vi "I2C_Download.vi"(11 "newFlashFW":u8[](array[numeric])) -> ()   [LabVIEW 2016]
uses:
  Global variable.vi
panel:
  out "status":u8
  in  "cmd_std_header_t":T1
  in  "执行部分":T2(ring)
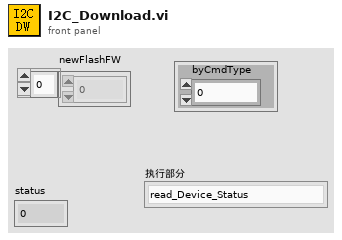
[diagram p1: front panel]
types:
  T1 = cluster{"byCmdType":u8, "bySubCmd":u8, "byPara":u8, "byAddr_h":u8, "byAddr_l":u8, "byAddr_ll":u8, "byLen_h":u8, "byLen_l":u8}
  T2 = enum16{"read_Device_Status", "RST_2_updateFW", "read_flashID_and_reset_flash", "erase_flash", "erase_check", "update_flashFW", "read_and_check", "write_Cache_TAG", "RST_2_ROM_and_check"}
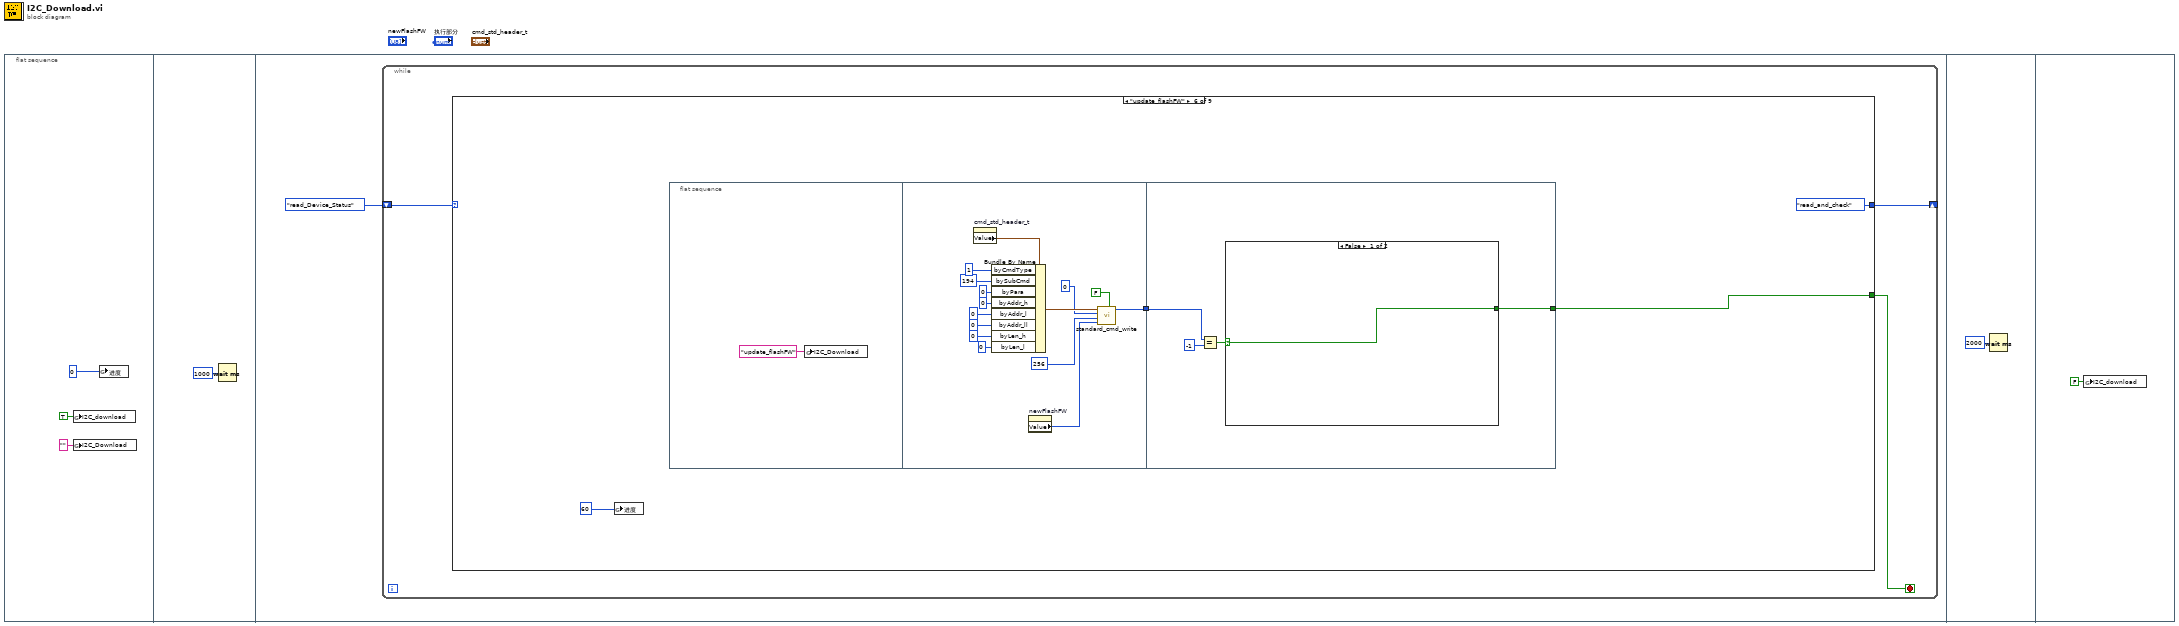
[diagram p0: block diagram]
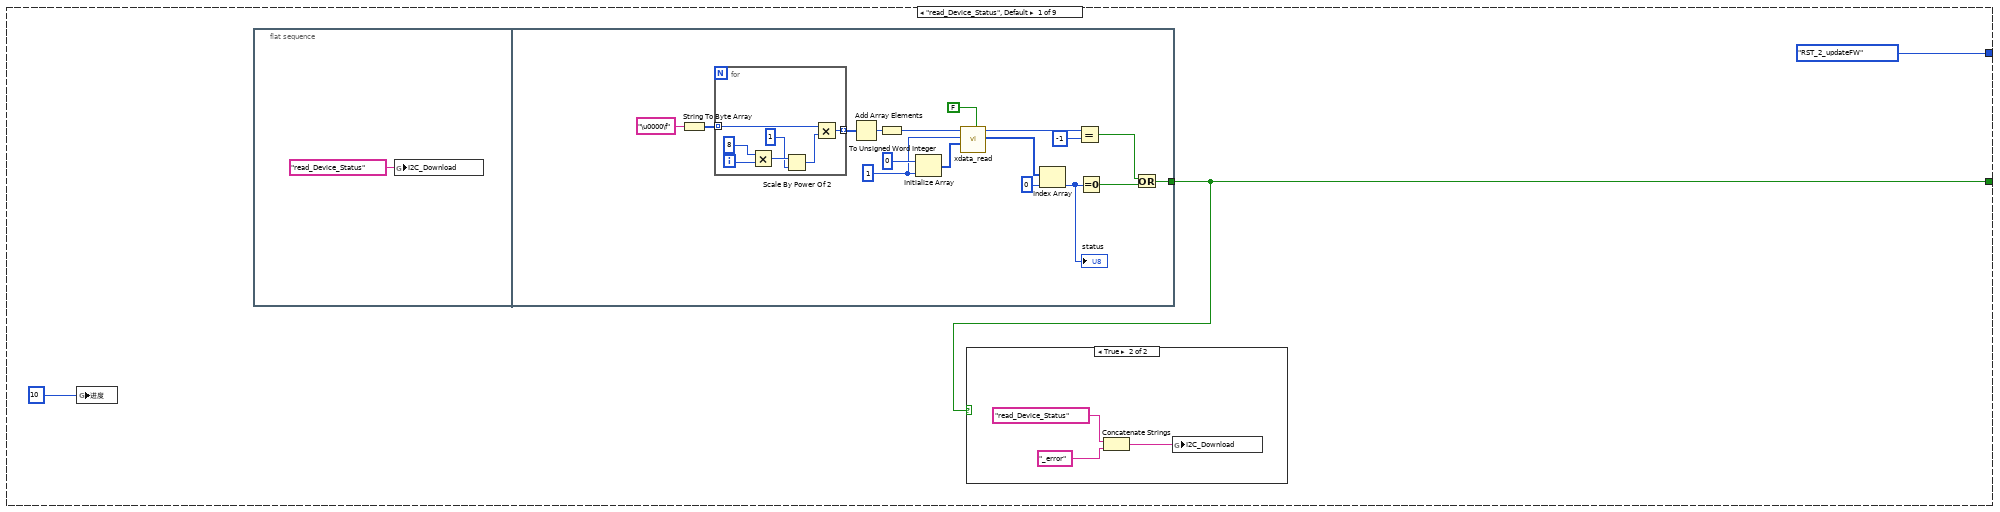
[diagram p2: hidden frame]
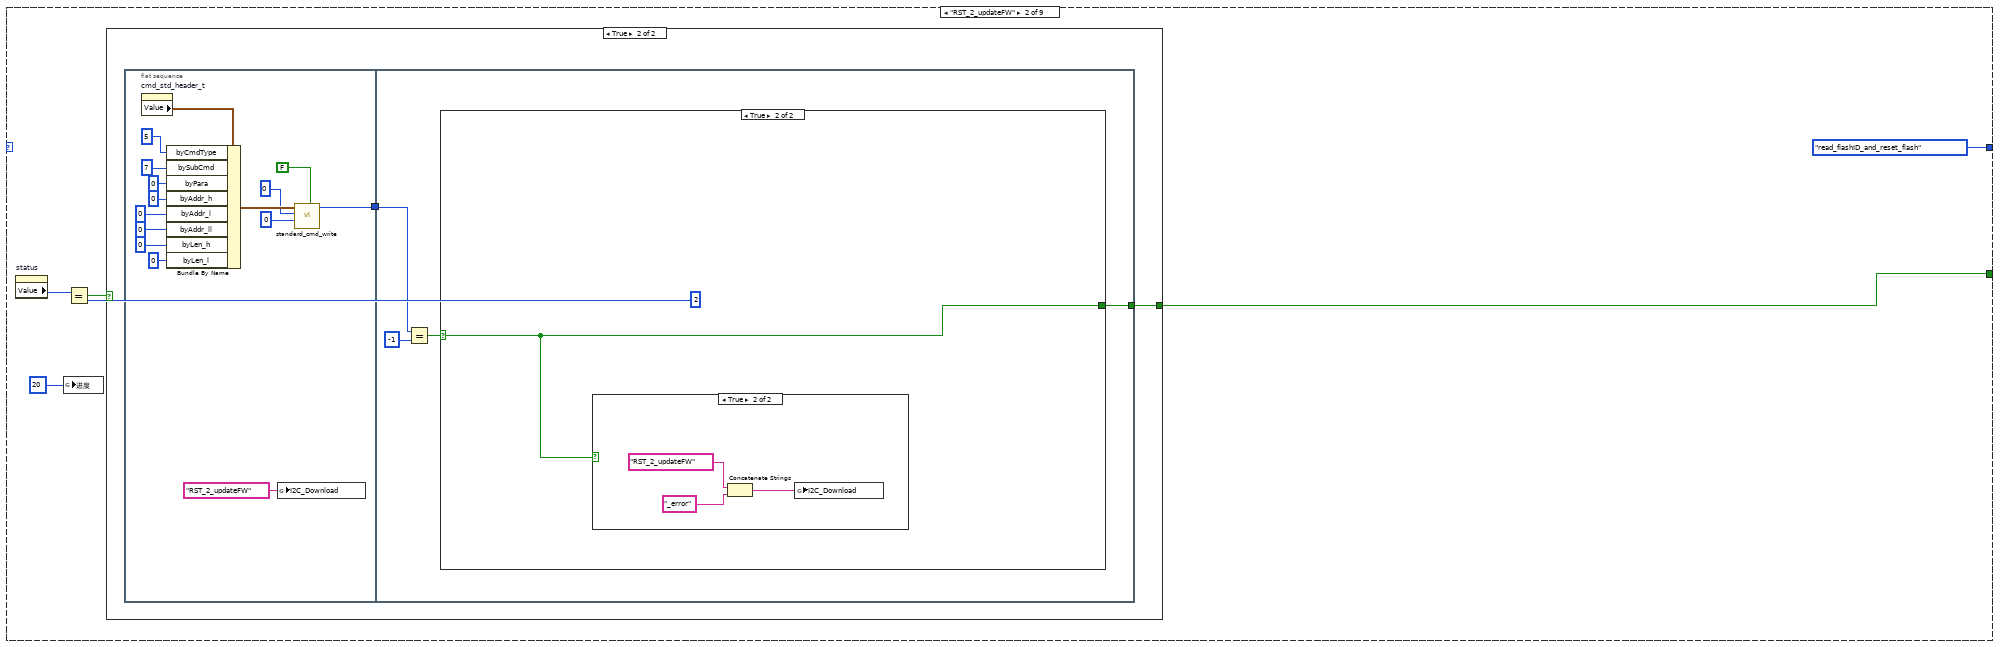
[diagram p4: hidden frame]
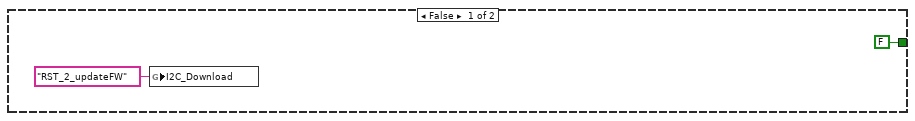
[diagram p5: hidden frame]
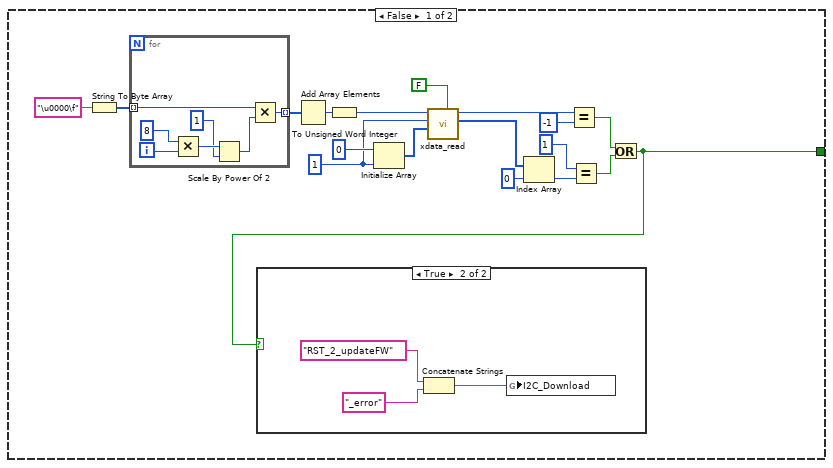
[diagram p6: hidden frame]
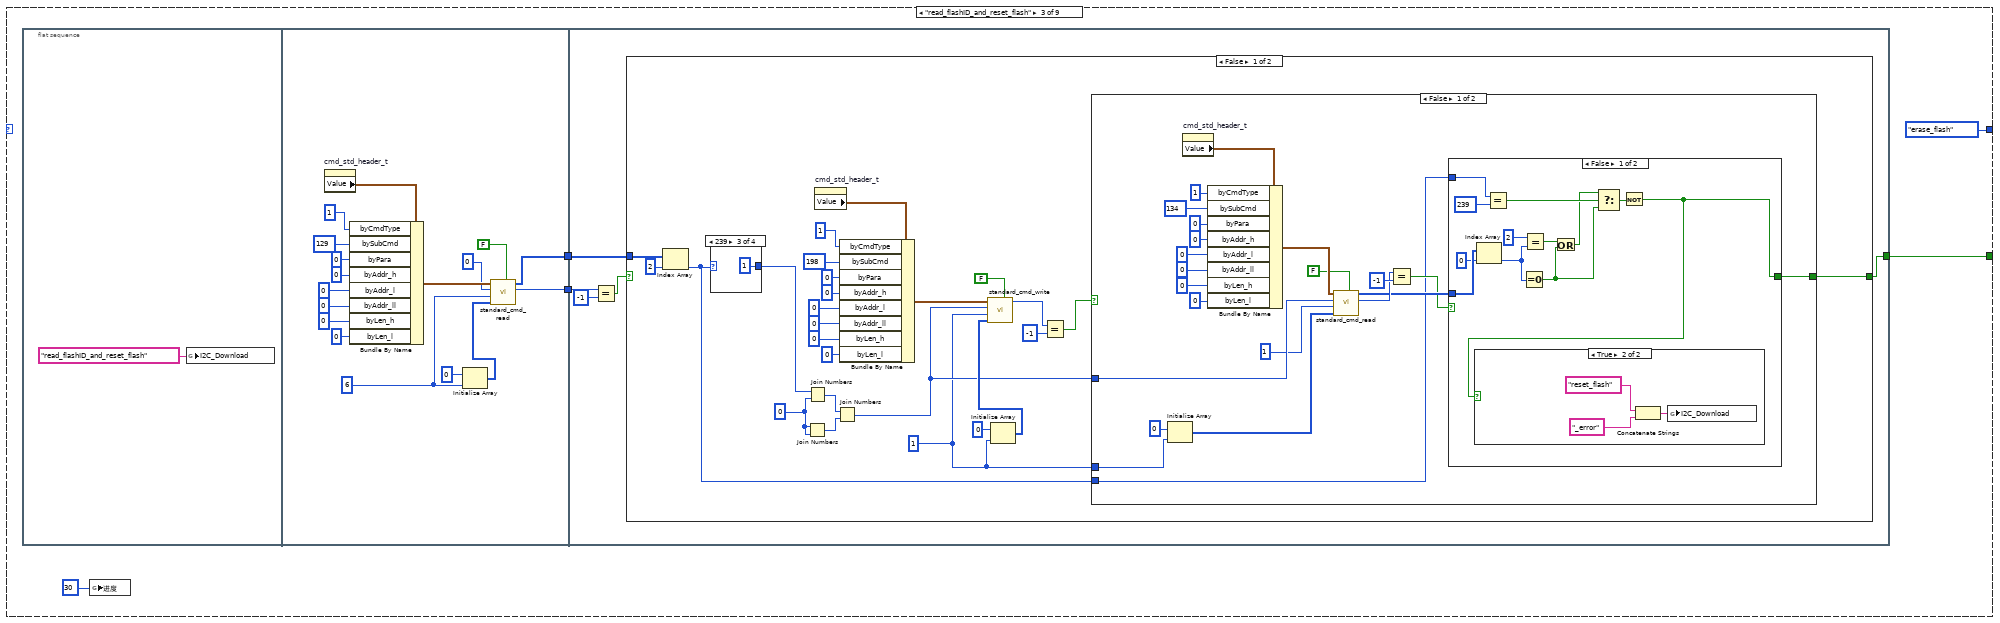
[diagram p9: hidden frame]
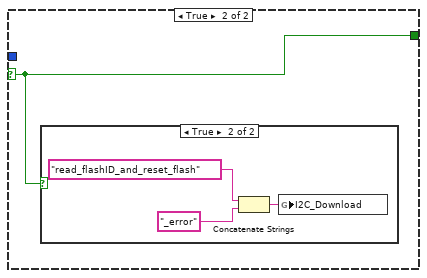
[diagram p11: hidden frame]
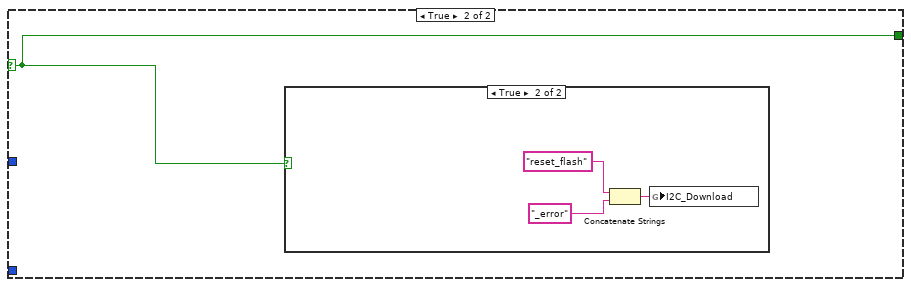
[diagram p13: hidden frame]
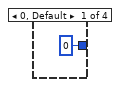
[diagram p15: hidden frame]
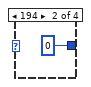
[diagram p16: hidden frame]
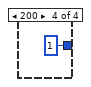
[diagram p17: hidden frame]
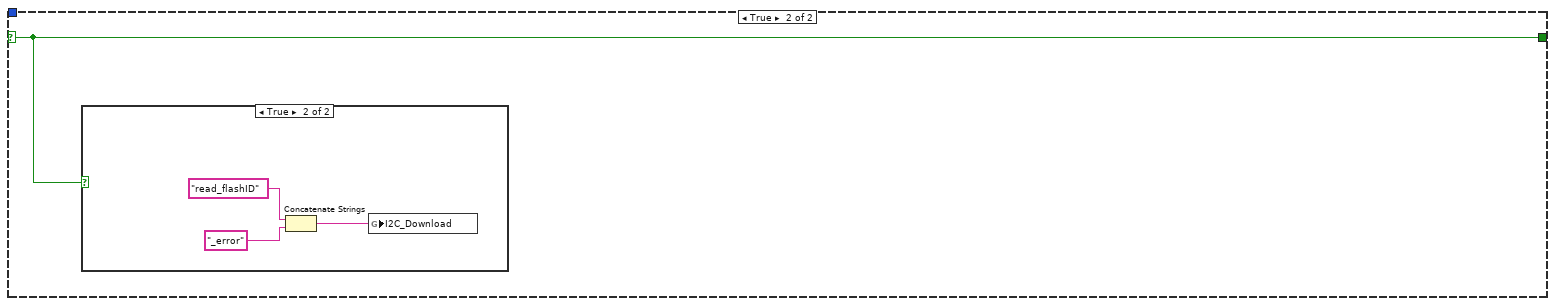
[diagram p18: hidden frame]
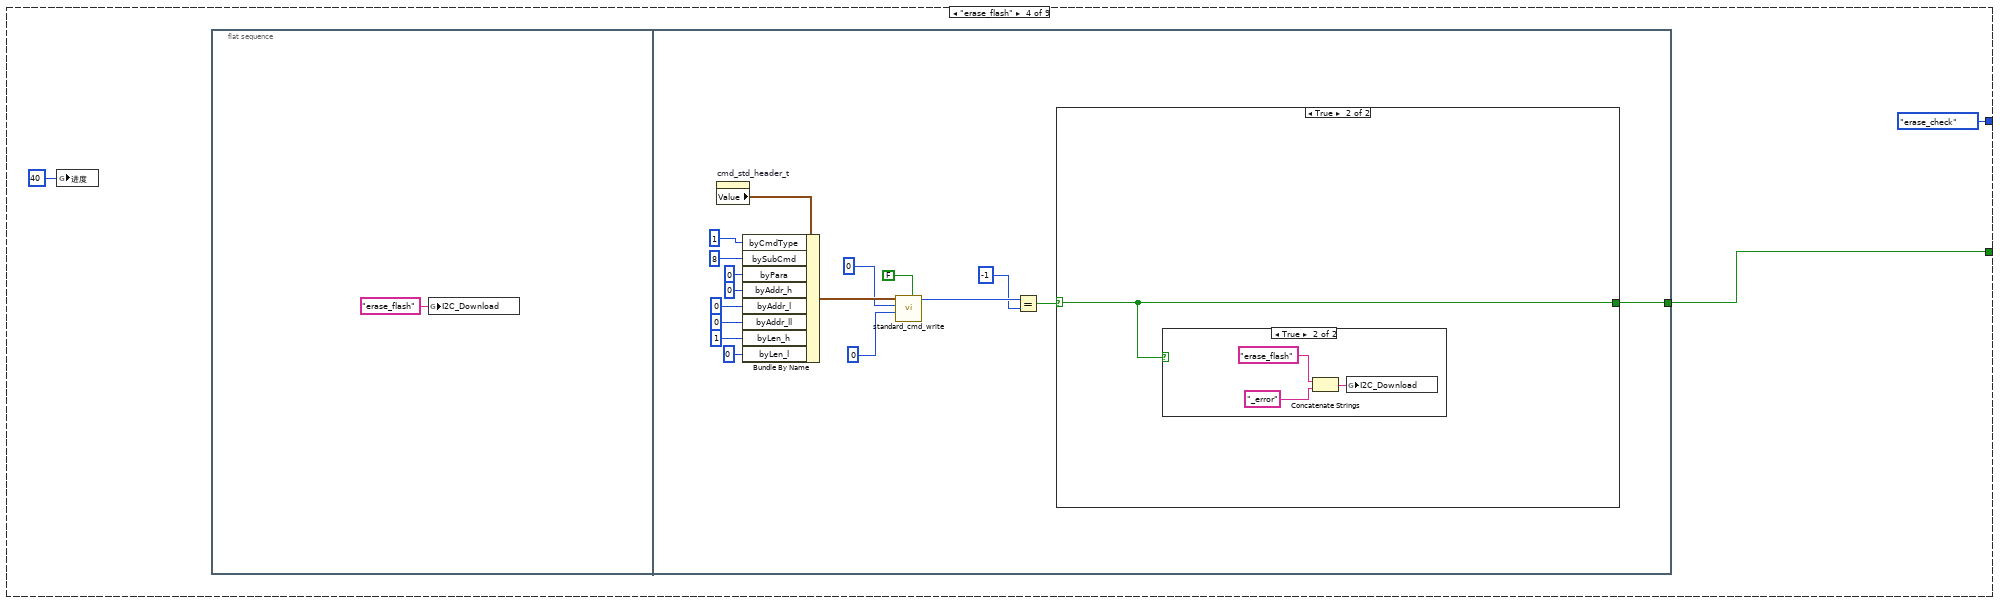
[diagram p20: hidden frame]
diagram:
  n1 = flat-sequence {
    frame #0 {
      n2 = global write "Global variable.vi" "I2C_download"(TRUE ("I2C_download")) -> ()
      n3 = global write "Global variable.vi" "I2C_Download"("" ("I2C_Download")) -> ()
      n4 = global write "Global variable.vi" "进度"(u8 0 ("进度")) -> ()
    }
    frame #1 {
      n5 = Wait (ms)(milliseconds to wait=u32 1000) -> ()  [unwired: 1 out]
    }
    frame #2 {
      n6 = while {
        shift-right: [w7] -> _
        shift-left: T2."read_Device_Status" ("执行部分") -> [w8]
        stop <- w6 stop-if-true
        n7 = case shown="\"update_flashFW\"" w8 {
          tunnel: [T2."RST_2_updateFW" ("执行部分") T2."read_flashID_and_reset_flash" ("执行部分") T2."erase_flash" ("执行部分") T2."erase_check" ("执行部分") T2."update_flashFW" ("执行部分") T2."read_and_check" ("执行部分") T2."write_Cache_TAG" ("执行部分") T2."RST_2_ROM_and_check" ("执行部分") T2."read_Device_Status" ("执行部分")] -> w7
          tunnel: [w10 w41 w102 w210 w236 w310 w339 w383 w411] -> w6
          frame "read_Device_Status", Default {
            n8 = global write "Global variable.vi" "进度"(u8 10 ("进度")) -> ()
            n9 = flat-sequence {
              tunnel: [w16] -> w10
              frame #0 {
                n10 = global write "Global variable.vi" "I2C_Download"("read_Device_Status" ("I2C_Download")) -> ()
              }
              frame #1 {
                w25 = 1 ("dimension size")
                n11 = String To Byte Array(string="\u0000\f") -> (unsigned byte array=w31:u8[])
                n12 = for {
                  tunnel: w31 -> [w34] mode=indexing
                  tunnel: [w33] -> w29 mode=indexing
                  i -> [w39]
                  n13 = Multiply(x=8, y=w39) -> (x*y=w37:i32)
                  n14 = Scale By Power Of 2(n=w37, x=1 ("x*y")) -> (x*2^n=w35:i32)
                  n15 = Multiply(x=w34, y=w35) -> (x*y=w33:i32)
                }
                n16 = Add Array Elements(numeric array=w29) -> (sum=w32:i32)
                n17 = To Unsigned Word Integer(number=w32) -> (unsigned 16bit integer=w28:u16)
                n18 = Initialize Array(u8 0 ("element"), w25) -> (w26:u8[])
                n19 = call "xdata_read.vi"("COM"=FALSE, "data"=w26, "wLen"=w25, "wAddr"=w28) -> ("data out"=w23:u8[], "return"=w20:i32)  [unwired: 6 in]
                n20 = Index Array(array=w23, index=0) -> (element=w21:u8)
                "status" <- w21
                n21 = Equal?(x=w20, y=-1) -> (x = y?=w18:bool)
                n22 = Equal To 0?(x=w21) -> (x = 0?=w17:bool)
                n23 = Or(x=w18, y=w17) -> (x .or. y?=w16:bool)
              }
            }
            n24 = case shown="True" w10 {
              frame False {
              }
              frame True {
                n25 = Concatenate Strings("read_Device_Status" ("I2C_Download"), "_error" ("I2C_Download")) -> (w12:string)
                n26 = global write "Global variable.vi" "I2C_Download"(w12) -> ()
              }
            }
          }
          frame "RST_2_updateFW" {
            n27 = property on="status" class="DigNum (strict)"() -> ("Value"=w45:u8)  [unwired: 2 in, 2 out]
            n28 = global write "Global variable.vi" "进度"(u8 20 ("进度")) -> ()
            n29 = Equal?(x=w45, y=u8 2) -> (x = y?=w43:bool)
            n30 = case shown="True" w43 {
              tunnel: [FALSE w48] -> w41
              frame False {
                n31 = global write "Global variable.vi" "I2C_Download"("RST_2_updateFW" ("I2C_Download")) -> ()
              }
              frame True {
                n32 = flat-sequence {
                  tunnel: [w51] -> w49
                  tunnel: w49 -> [w67]
                  tunnel: [w65] -> w48
                  frame #0 {
                    n33 = property on="cmd_std_header_t" class="Clust (strict)"() -> ("Value"=w64:T1)  [unwired: 2 in, 2 out]
                    n34 = Bundle By Name(cluster=w64, "byCmdType"=u8 5, "bySubCmd"=u8 7, "byPara"=u8 0, "byAddr_h"=u8 0, "byAddr_l"=u8 0, "byAddr_ll"=u8 0, "byLen_h"=u8 0, "byLen_l"=u8 0) -> (w55:T1)
                    n35 = global write "Global variable.vi" "I2C_Download"("RST_2_updateFW" ("I2C_Download")) -> ()
                    n36 = call "standard_cmd_write.vi"("COM"=FALSE, "dwLen"=u32 0, "dwAddr"=u32 0, "cmd_std_header_t"=w55) -> ("return"=w51:i32)  [unwired: 7 in]
                  }
                  frame #1 {
                    n37 = Equal?(x=w67, y=-1) -> (x = y?=w68:bool)
                    n38 = case shown="True" w68 {
                      selector: w68 -> [_ w97]
                      tunnel: [w70 w97] -> w65
                      frame False {
                        w79 = 1 ("dimension size")
                        n39 = String To Byte Array(string="\u0000\f") -> (unsigned byte array=w85:u8[])
                        n40 = for {
                          tunnel: w85 -> [w91] mode=indexing
                          tunnel: [w90] -> w83 mode=indexing
                          i -> [w96]
                          n41 = Multiply(x=8, y=w96) -> (x*y=w94:i32)
                          n42 = Scale By Power Of 2(n=w94, x=1 ("x*y")) -> (x*2^n=w92:i32)
                          n43 = Multiply(x=w91, y=w92) -> (x*y=w90:i32)
                        }
                        n44 = Add Array Elements(numeric array=w83) -> (sum=w86:i32)
                        n45 = To Unsigned Word Integer(number=w86) -> (unsigned 16bit integer=w82:u16)
                        n46 = Initialize Array(u8 0 ("element"), w79) -> (w80:u8[])
                        n47 = call "xdata_read.vi"("COM"=FALSE, "data"=w80, "wLen"=w79, "wAddr"=w82) -> ("data out"=w77:u8[], "return"=w74:i32)  [unwired: 6 in]
                        n48 = Index Array(array=w77, index=0) -> (element=w75:u8)
                        n49 = Equal?(x=w74, y=-1) -> (x = y?=w72:bool)
                        n50 = Equal?(x=u8 1, y=w75) -> (x = y?=w71:bool)
                        n51 = Or(x=w72, y=w71) -> (x .or. y?=w70:bool)
                        n52 = case shown="True" w70 {
                          frame False {
                          }
                          frame True {
                            n53 = Concatenate Strings("RST_2_updateFW" ("I2C_Download"), "_error" ("I2C_Download")) -> (w87:string)
                            n54 = global write "Global variable.vi" "I2C_Download"(w87) -> ()
                          }
                        }
                      }
                      frame True {
                        n55 = case shown="True" w97 {
                          frame False {
                          }
                          frame True {
                            n56 = Concatenate Strings("RST_2_updateFW" ("I2C_Download"), "_error" ("I2C_Download")) -> (w98:string)
                            n57 = global write "Global variable.vi" "I2C_Download"(w98) -> ()
                          }
                        }
                      }
                    }
                  }
                }
              }
            }
          }
          frame "read_flashID_and_reset_flash" {
            n58 = flat-sequence {
              tunnel: [w108] -> w105
              tunnel: [w107] -> w104
              tunnel: w105 -> [w128]
              tunnel: w104 -> [w124]
              tunnel: [w125] -> w102
              frame #0 {
                n59 = global write "Global variable.vi" "I2C_Download"("read_flashID_and_reset_flash" ("I2C_Download")) -> ()
              }
              frame #1 {
                w112 = u32 6 ("dwLen")
                n60 = property on="cmd_std_header_t" class="Clust (strict)"() -> ("Value"=w123:T1)  [unwired: 2 in, 2 out]
                n61 = Bundle By Name(cluster=w123, "byCmdType"=u8 1, "bySubCmd"=u8 129, "byPara"=u8 0, "byAddr_h"=u8 0, "byAddr_l"=u8 0, "byAddr_ll"=u8 0, "byLen_h"=u8 0, "byLen_l"=u8 0) -> (w114:T1)
                n62 = Initialize Array(u8 0 ("element"), w112) -> (w111:u8[])
                n63 = call "standard_cmd_read.vi"("COM"=FALSE, "data"=w111, "dwLen"=w112, "dwAddr"=u32 0, "cmd_std_header_t"=w114) -> ("return"=w108:i32, "data out"=w107:u8[])  [unwired: 5 in]
              }
              frame #2 {
                n64 = Equal?(x=w128, y=-1) -> (x = y?=w126:bool)
                n65 = case shown="False" w126 {
                  selector: w126 -> [_ w204]
                  tunnel: [w130 w204] -> w125
                  tunnel: w124 -> [w154 _]
                  frame False {
                    w131 = u32 1 ("dwLen")
                    w140 = u8 0 ("element")
                    n66 = Index Array(array=w154, index=2) -> (element=w129:u8)
                    n67 = case shown="239" w129 {
                      tunnel: [u8 0 ("element") u8 0 ("element") u8 1 ("element") u8 1 ("element")] -> w133
                      frame 0, Default {
                      }
                      frame 194 {
                      }
                      frame 239 {
                      }
                      frame 200 {
                      }
                    }
                    n68 = Join Numbers(hi=w140, lo=w140) -> ((hi.lo)=w142:u16)
                    n69 = Join Numbers(hi=w133, lo=w140) -> ((hi.lo)=w141:u16)
                    n70 = property on="cmd_std_header_t" class="Clust (strict)"() -> ("Value"=w144:T1)  [unwired: 2 in, 2 out]
                    n71 = Join Numbers(hi=w141, lo=w142) -> ((hi.lo)=w132:u32)
                    n72 = Bundle By Name(cluster=w144, "byCmdType"=u8 1, "bySubCmd"=u8 198, "byPara"=u8 0, "byAddr_h"=u8 0, "byAddr_l"=u8 0, "byAddr_ll"=u8 0, "byLen_h"=u8 0, "byLen_l"=u8 0) -> (w143:T1)
                    n73 = Initialize Array(u8 0 ("element"), w131) -> (w138:u8[])
                    n74 = call "standard_cmd_write.vi"("COM"=FALSE, "data"=w138, "dwLen"=w131, "dwAddr"=w132, "cmd_std_header_t"=w143) -> ("return"=w135:i32)  [unwired: 6 in]
                    n75 = Equal?(x=w135, y=-1) -> (x = y?=w134:bool)
                    n76 = case shown="False" w134 {
                      selector: w134 -> [_ w196]
                      tunnel: w132 -> [w166 _]
                      tunnel: w131 -> [w163 _]
                      tunnel: [w156 w196] -> w130
                      tunnel: w129 -> [w155 _]
                      frame False {
                        n77 = Initialize Array(u8 0 ("element"), w163) -> (w162:u8[])
                        n78 = property on="cmd_std_header_t" class="Clust (strict)"() -> ("Value"=w176:T1)  [unwired: 2 in, 2 out]
                        n79 = Bundle By Name(cluster=w176, "byCmdType"=u8 1, "bySubCmd"=u8 134, "byPara"=u8 0, "byAddr_h"=u8 0, "byAddr_l"=u8 0, "byAddr_ll"=u8 0, "byLen_h"=u8 0, "byLen_l"=u8 0) -> (w167:T1)
                        n80 = call "standard_cmd_read.vi"("COM"=FALSE, "data"=w162, "dwLen"=u32 1, "dwAddr"=w166, "cmd_std_header_t"=w167) -> ("return"=w159:i32, "data out"=w158:u8[])  [unwired: 5 in]
                        n81 = Equal?(x=w159, y=-1) -> (x = y?=w157:bool)
                        n82 = case shown="False" w157 {
                          selector: w157 -> [_ w192]
                          tunnel: w158 -> [w188 _]
                          tunnel: [w177 w192] -> w156
                          tunnel: w155 -> [w186 _]
                          frame False {
                            n83 = Index Array(array=w188, index=0) -> (element=w184:u8)
                            n84 = Equal?(x=w186, y=u8 239) -> (x = y?=w181:bool)
                            n85 = Equal To 0?(x=w184) -> (x = 0?=w179:bool)
                            n86 = Equal?(x=u8 2, y=w184) -> (x = y?=w182:bool)
                            n87 = Or(x=w182, y=w179) -> (x .or. y?=w180:bool)
                            n88 = Select(t=w180, s=w181, f=w179) -> (s? t:f=w178:bool)
                            n89 = Not(x=w178) -> (.not. x?=w177:bool)
                            n90 = case shown="True" w177 {
                              frame False {
                              }
                              frame True {
                                n91 = Concatenate Strings("reset_flash" ("I2C_Download"), "_error" ("I2C_Download")) -> (w189:string)
                                n92 = global write "Global variable.vi" "I2C_Download"(w189) -> ()
                              }
                            }
                          }
                          frame True {
                            n93 = case shown="True" w192 {
                              frame False {
                              }
                              frame True {
                                n94 = Concatenate Strings("read_flashID_and_reset_flash" ("I2C_Download"), "_error" ("I2C_Download")) -> (w193:string)
                                n95 = global write "Global variable.vi" "I2C_Download"(w193) -> ()
                              }
                            }
                          }
                        }
                      }
                      frame True {
                        n96 = case shown="True" w196 {
                          frame False {
                          }
                          frame True {
                            n97 = Concatenate Strings("reset_flash" ("I2C_Download"), "_error" ("I2C_Download")) -> (w197:string)
                            n98 = global write "Global variable.vi" "I2C_Download"(w197) -> ()
                          }
                        }
                      }
                    }
                  }
                  frame True {
                    n99 = case shown="True" w204 {
                      frame False {
                      }
                      frame True {
                        n100 = Concatenate Strings("read_flashID" ("I2C_Download"), "_error" ("I2C_Download")) -> (w205:string)
                        n101 = global write "Global variable.vi" "I2C_Download"(w205) -> ()
                      }
                    }
                  }
                }
              }
            }
            n102 = global write "Global variable.vi" "进度"(u8 30 ("进度")) -> ()
          }
          frame "erase_flash" {
            n103 = global write "Global variable.vi" "进度"(u8 40 ("进度")) -> ()
            n104 = flat-sequence {
              tunnel: [w212] -> w210
              frame #0 {
                n105 = global write "Global variable.vi" "I2C_Download"("erase_flash" ("I2C_Download")) -> ()
              }
              frame #1 {
                n106 = property on="cmd_std_header_t" class="Clust (strict)"() -> ("Value"=w228:T1)  [unwired: 2 in, 2 out]
                n107 = Bundle By Name(cluster=w228, "byCmdType"=u8 1, "bySubCmd"=u8 8, "byPara"=u8 0, "byAddr_h"=u8 0, "byAddr_l"=u8 0, "byAddr_ll"=u8 0, "byLen_h"=u8 1, "byLen_l"=u8 0) -> (w227:T1)
                n108 = call "standard_cmd_write.vi"("COM"=FALSE, "dwLen"=u32 0, "dwAddr"=u32 0, "cmd_std_header_t"=w227) -> ("return"=w215:i32)  [unwired: 7 in]
                n109 = Equal?(x=w215, y=-1) -> (x = y?=w213:bool)
                n110 = case shown="True" w213 {
                  selector: w213 -> [w229 w230]
                  tunnel: [w229 w230] -> w212
                  frame False {
                  }
                  frame True {
                    n111 = case shown="True" w230 {
                      frame False {
                      }
                      frame True {
                        n112 = Concatenate Strings("erase_flash" ("I2C_Download"), "_error" ("I2C_Download")) -> (w231:string)
                        n113 = global write "Global variable.vi" "I2C_Download"(w231) -> ()
                      }
                    }
                  }
                }
              }
            }
          }
          frame "erase_check" {
            n114 = global write "Global variable.vi" "进度"(u8 50 ("进度")) -> ()
            n115 = flat-sequence {
              tunnel: [w245] -> w241
              tunnel: [w244] -> w237
              tunnel: [w264] -> w242
              tunnel: w241 -> [w264]
              tunnel: [w263] -> w240
              tunnel: [w262] -> w239
              tunnel: [w261] -> w238
              tunnel: w237 -> [w261]
              tunnel: w242 -> [w293]
              tunnel: w240 -> [w296]
              tunnel: [w289] -> w236
              tunnel: w239 -> [w285]
              tunnel: w238 -> [w288]
              frame #0 {
                n116 = global write "Global variable.vi" "I2C_Download"("erase_check" ("I2C_Download")) -> ()
              }
              frame #1 {
                w248 = u32 4096 ("dwLen")
                n117 = property on="cmd_std_header_t" class="Clust (strict)"() -> ("Value"=w259:T1)  [unwired: 2 in, 2 out]
                n118 = Bundle By Name(cluster=w259, "byCmdType"=u8 1, "bySubCmd"=u8 130, "byPara"=u8 0, "byAddr_h"=u8 0, "byAddr_l"=u8 0, "byAddr_ll"=u8 0, "byLen_h"=u8 0, "byLen_l"=u8 0) -> (w260:T1)
                n119 = Initialize Array(u8 0 ("element"), w248) -> (w247:u8[])
                n120 = call "standard_cmd_read.vi"("COM"=FALSE, "data"=w247, "dwLen"=w248, "dwAddr"=u32 0, "cmd_std_header_t"=w260) -> ("return"=w245:i32, "data out"=w244:u8[])  [unwired: 5 in]
              }
              frame #2 {
                w277 = u32 4096 ("dwLen")
                n121 = property on="cmd_std_header_t" class="Clust (strict)"() -> ("Value"=w266:T1)  [unwired: 2 in, 2 out]
                n122 = Bundle By Name(cluster=w266, "byCmdType"=u8 1, "bySubCmd"=u8 130, "byPara"=u8 0, "byAddr_h"=u8 0, "byAddr_l"=u8 0, "byAddr_ll"=u8 0, "byLen_h"=u8 0, "byLen_l"=u8 0) -> (w265:T1)
                n123 = Initialize Array(u8 0 ("element"), w277) -> (w278:u8[])
                n124 = call "standard_cmd_read.vi"("COM"=FALSE, "data"=w278, "dwLen"=w277, "dwAddr"=u32 258048, "cmd_std_header_t"=w265) -> ("return"=w263:i32, "data out"=w262:u8[])  [unwired: 5 in]
              }
              frame #3 {
                n125 = Equal?(x=w296, y=-1) -> (x = y?=w292:bool)
                n126 = Equal?(x=w293, y=-1) -> (x = y?=w291:bool)
                n127 = Equal?(x=u8 255 ("y"), y=w288) -> (x = y?=w284:bool[])
                n128 = Equal?(x=w285, y=u8 255) -> (x = y?=w283:bool[])
                n129 = Or(x=w292, y=w291) -> (x .or. y?=w290:bool)
                n130 = And Array Elements(Boolean array=w284) -> (logical AND=w281:bool)
                n131 = And Array Elements(Boolean array=w283) -> (logical AND=w282:bool)
                n132 = And(x=w281, y=w282) -> (x .and. y?=w280:bool)
                n133 = case shown="False" w290 {
                  selector: w290 -> [_ w304]
                  tunnel: [w297 w304] -> w289
                  tunnel: w280 -> [w298 _]
                  frame False {
                    n134 = case shown="False" w298 {
                      tunnel: [w299 FALSE] -> w297
                      frame False {
                        w299 = TRUE
                        n135 = case shown="True" w299 {
                          frame False {
                          }
                          frame True {
                            n136 = Concatenate Strings("erase_check" ("I2C_Download"), "_error" ("I2C_Download")) -> (w300:string)
                            n137 = global write "Global variable.vi" "I2C_Download"(w300) -> ()
                          }
                        }
                      }
                      frame True {
                      }
                    }
                  }
                  frame True {
                    n138 = case shown="True" w304 {
                      frame False {
                      }
                      frame True {
                        n139 = Concatenate Strings("erase_check" ("I2C_Download"), "_error" ("I2C_Download")) -> (w305:string)
                        n140 = global write "Global variable.vi" "I2C_Download"(w305) -> ()
                      }
                    }
                  }
                }
              }
            }
          }
          frame "update_flashFW" {
            n141 = global write "Global variable.vi" "进度"(u8 60 ("进度")) -> ()
            n142 = flat-sequence {
              tunnel: [w314] -> w311
              tunnel: w311 -> [w330]
              tunnel: [w328] -> w310
              frame #0 {
                n143 = global write "Global variable.vi" "I2C_Download"("update_flashFW" ("I2C_Download")) -> ()
              }
              frame #1 {
                n144 = property on="cmd_std_header_t" class="Clust (strict)"() -> ("Value"=w327:T1)  [unwired: 2 in, 2 out]
                n145 = Bundle By Name(cluster=w327, "byCmdType"=u8 1, "bySubCmd"=u8 194, "byPara"=u8 0, "byAddr_h"=u8 0, "byAddr_l"=u8 0, "byAddr_ll"=u8 0, "byLen_h"=u8 0, "byLen_l"=u8 0) -> (w326:T1)
                n146 = property on="newFlashFW" class="Arr (strict)"() -> ("Value"=w313:u8[])  [unwired: 2 in, 2 out]
                n147 = call "standard_cmd_write.vi"("COM"=FALSE, "data"=w313, "dwLen"=u32 256, "dwAddr"=u32 0, "cmd_std_header_t"=w326) -> ("return"=w314:i32)  [unwired: 6 in]
              }
              frame #2 {
                n148 = Equal?(x=w330, y=-1) -> (x = y?=w331:bool)
                n149 = case shown="False" w331 {
                  selector: w331 -> [w332 w333]
                  tunnel: [w332 w333] -> w328
                  frame False {
                  }
                  frame True {
                    n150 = case shown="True" w333 {
                      frame False {
                      }
                      frame True {
                        n151 = Concatenate Strings("update_flashFW" ("I2C_Download"), "_error" ("I2C_Download")) -> (w334:string)
                        n152 = global write "Global variable.vi" "I2C_Download"(w334) -> ()
                      }
                    }
                  }
                }
              }
            }
          }
          frame "read_and_check" {
            n153 = global write "Global variable.vi" "进度"(u8 70 ("进度")) -> ()
            n154 = flat-sequence {
              tunnel: [w348] -> w341
              tunnel: [w343] -> w340
              tunnel: w341 -> [w363]
              tunnel: [w361] -> w339
              tunnel: w340 -> [w360]
              frame #0 {
                n155 = global write "Global variable.vi" "I2C_Download"("read_and_check" ("I2C_Download")) -> ()
              }
              frame #1 {
                w345 = u32 256 ("dwLen")
                n156 = property on="cmd_std_header_t" class="Clust (strict)"() -> ("Value"=w347:T1)  [unwired: 2 in, 2 out]
                n157 = Bundle By Name(cluster=w347, "byCmdType"=u8 1, "bySubCmd"=u8 130, "byPara"=u8 0, "byAddr_h"=u8 0, "byAddr_l"=u8 0, "byAddr_ll"=u8 0, "byLen_h"=u8 0, "byLen_l"=u8 0) -> (w359:T1)
                n158 = Initialize Array(u8 0 ("element"), w345) -> (w344:u8[])
                n159 = call "standard_cmd_read.vi"("COM"=FALSE, "data"=w344, "dwLen"=w345, "dwAddr"=u32 0, "cmd_std_header_t"=w359) -> ("return"=w348:i32, "data out"=w343:u8[])  [unwired: 5 in]
              }
              frame #2 {
                n160 = Equal?(x=w363, y=-1) -> (x = y?=w364:bool)
                n161 = case shown="False" w364 {
                  selector: w364 -> [_ w377]
                  tunnel: [w365 w377] -> w361
                  tunnel: w360 -> [w369 _]
                  frame False {
                    n162 = property on="newFlashFW" class="Arr (strict)"() -> ("Value"=w368:u8[])  [unwired: 2 in, 2 out]
                    n163 = Equal?(x=w369, y=w368) -> (x = y?=w367:bool[])
                    n164 = And Array Elements(Boolean array=w367) -> (logical AND=w366:bool)
                    n165 = case shown="False" w366 {
                      selector: w366 -> [w371 w376]
                      tunnel: [w370 w375] -> w365
                      frame False {
                        n166 = Not(x=w371) -> (.not. x?=w370:bool)
                        n167 = case shown="True" w370 {
                          frame False {
                          }
                          frame True {
                            n168 = Concatenate Strings("read_and_check" ("I2C_Download"), "_error" ("I2C_Download")) -> (w372:string)
                            n169 = global write "Global variable.vi" "I2C_Download"(w372) -> ()
                          }
                        }
                      }
                      frame True {
                        n170 = Not(x=w376) -> (.not. x?=w375:bool)
                      }
                    }
                  }
                  frame True {
                    n171 = case shown="True" w377 {
                      frame False {
                      }
                      frame True {
                        n172 = Concatenate Strings("update_flashFW" ("I2C_Download"), "_error" ("I2C_Download")) -> (w378:string)
                        n173 = global write "Global variable.vi" "I2C_Download"(w378) -> ()
                      }
                    }
                  }
                }
              }
            }
          }
          frame "write_Cache_TAG" {
            n174 = global write "Global variable.vi" "进度"(u8 80 ("进度")) -> ()
            n175 = flat-sequence {
              tunnel: [w386] -> w384
              tunnel: w384 -> [w402]
              tunnel: [w400] -> w383
              frame #0 {
                n176 = global write "Global variable.vi" "I2C_Download"("write_Cache_TAG" ("I2C_Download")) -> ()
              }
              frame #1 {
                n177 = property on="cmd_std_header_t" class="Clust (strict)"() -> ("Value"=w399:T1)  [unwired: 2 in, 2 out]
                n178 = Bundle By Name(cluster=w399, "byCmdType"=u8 1, "bySubCmd"=u8 9, "byPara"=u8 0, "byAddr_h"=u8 0, "byAddr_l"=u8 0, "byAddr_ll"=u8 0, "byLen_h"=u8 0, "byLen_l"=u8 0) -> (w398:T1)
                n179 = call "standard_cmd_write.vi"("COM"=FALSE, "dwLen"=u32 0, "dwAddr"=u32 0, "cmd_std_header_t"=w398) -> ("return"=w386:i32)  [unwired: 7 in]
              }
              frame #2 {
                n180 = Equal?(x=w402, y=-1) -> (x = y?=w403:bool)
                n181 = case shown="True" w403 {
                  selector: w403 -> [w404 w405]
                  tunnel: [w404 w405] -> w400
                  frame False {
                  }
                  frame True {
                    n182 = case shown="True" w405 {
                      frame False {
                      }
                      frame True {
                        n183 = Concatenate Strings("write_Cache_TAG" ("I2C_Download"), "_error" ("I2C_Download")) -> (w406:string)
                        n184 = global write "Global variable.vi" "I2C_Download"(w406) -> ()
                      }
                    }
                  }
                }
              }
            }
          }
          frame "RST_2_ROM_and_check" {
            n185 = global write "Global variable.vi" "进度"(u8 90 ("进度")) -> ()
            n186 = flat-sequence {
              tunnel: [w415] -> w412
              tunnel: w412 -> [w430]
              tunnel: [w428] -> w411
              frame #0 {
                n187 = global write "Global variable.vi" "I2C_Download"("RST_2_ROM_and_check" ("I2C_Download")) -> ()
              }
              frame #1 {
                n188 = property on="cmd_std_header_t" class="Clust (strict)"() -> ("Value"=w414:T1)  [unwired: 2 in, 2 out]
                n189 = Bundle By Name(cluster=w414, "byCmdType"=u8 5, "bySubCmd"=u8 8, "byPara"=u8 0, "byAddr_h"=u8 0, "byAddr_l"=u8 0, "byAddr_ll"=u8 0, "byLen_h"=u8 0, "byLen_l"=u8 0) -> (w427:T1)
                n190 = call "standard_cmd_write.vi"("COM"=FALSE, "dwLen"=u32 0, "dwAddr"=u32 0, "cmd_std_header_t"=w427) -> ("return"=w415:i32)  [unwired: 7 in]
              }
              frame #2 {
                n191 = Equal?(x=w430, y=-1) -> (x = y?=w431:bool)
                n192 = case shown="False" w431 {
                  selector: w431 -> [_ w462]
                  tunnel: [TRUE TRUE] -> w428
                  frame False {
                    w442 = 1 ("dimension size")
                    n193 = String To Byte Array(string="\u0000\f") -> (unsigned byte array=w448:u8[])
                    n194 = for {
                      tunnel: w448 -> [w455] mode=indexing
                      tunnel: [w454] -> w446 mode=indexing
                      i -> [w460]
                      n195 = Multiply(x=8, y=w460) -> (x*y=w458:i32)
                      n196 = Scale By Power Of 2(n=w458, x=1 ("x*y")) -> (x*2^n=w456:i32)
                      n197 = Multiply(x=w455, y=w456) -> (x*y=w454:i32)
                    }
                    n198 = Add Array Elements(numeric array=w446) -> (sum=w449:i32)
                    n199 = To Unsigned Word Integer(number=w449) -> (unsigned 16bit integer=w445:u16)
                    n200 = Initialize Array(u8 0 ("element"), w442) -> (w443:u8[])
                    n201 = call "xdata_read.vi"("COM"=FALSE, "data"=w443, "wLen"=w442, "wAddr"=w445) -> ("data out"=w440:u8[], "return"=w437:i32)  [unwired: 6 in]
                    n202 = Index Array(array=w440, index=0) -> (element=w438:u8)
                    n203 = Equal?(x=w437, y=-1) -> (x = y?=w435:bool)
                    n204 = Equal To 0?(x=w438) -> (x = 0?=w434:bool)
                    n205 = Or(x=w435, y=w434) -> (x .or. y?=w433:bool)
                    n206 = case shown="False" w433 {
                      frame False {
                        n207 = global write "Global variable.vi" "进度"(u8 100 ("进度")) -> ()
                      }
                      frame True {
                        n208 = Concatenate Strings("RST_2_ROM_and_check" ("I2C_Download"), "_error" ("I2C_Download")) -> (w451:string)
                        n209 = global write "Global variable.vi" "I2C_Download"(w451) -> ()
                      }
                    }
                  }
                  frame True {
                    n210 = case shown="True" w462 {
                      frame False {
                      }
                      frame True {
                        n211 = Concatenate Strings("RST_2_ROM_and_check" ("I2C_Download"), "_error" ("I2C_Download")) -> (w463:string)
                        n212 = global write "Global variable.vi" "I2C_Download"(w463) -> ()
                      }
                    }
                  }
                }
              }
            }
          }
        }
      }
    }
    frame #3 {
      n213 = Wait (ms)(milliseconds to wait=u32 2000) -> ()  [unwired: 1 out]
    }
    frame #4 {
      n214 = global write "Global variable.vi" "I2C_download"(FALSE ("I2C_download")) -> ()
    }
  }
